vi "CRYPort Number Finder.vi"(9 "N interfs":i32=3, 10 "Interf settings":T1(array[cluster]), 11 "RS-232 type":enum16{"comm", "footswitch", "buzzer"}(ring)) -> (2 "Such a port exists":bool, 3 "Port (LV)":i32)   [LabVIEW 2013]
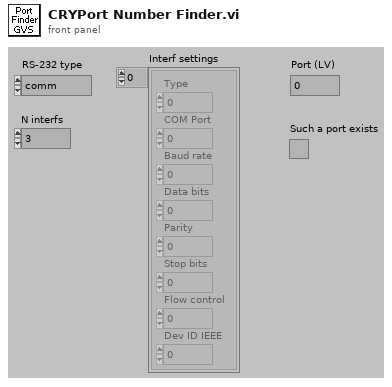
[diagram p1: front panel]
types:
  T1 = cluster{"Type":u16, "COM Port":u8, "Baud rate":u32, "Data bits":u32, "Parity":u16, "Stop bits":u16, "Flow control":u16, "Dev ID IEEE":u8}[]
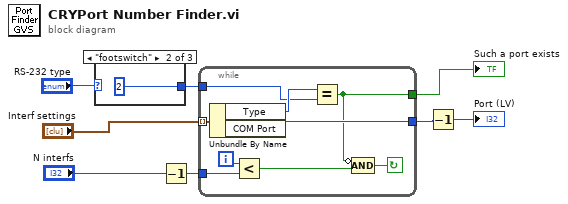
[diagram p0: block diagram]
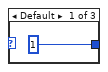
[diagram p2: hidden frame]
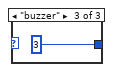
[diagram p3: hidden frame]
diagram:
  n1 = case shown="\"footswitch\"" "RS-232 type" {
    tunnel: [1 2 3] -> w6
    frame Default {
    }
    frame "footswitch" {
    }
    frame "buzzer" {
    }
  }
  n2 = Decrement(x="N interfs") -> (x-1=w8:i32)
  n3 = while {
    tunnel: w6 -> [w12]
    tunnel: [w13] -> w3
    tunnel: [w14] -> w2
    tunnel: w8 -> [w20]
    tunnel: "Interf settings" -> [w16] mode=indexing
    i -> [w19]
    stop <- w15 continue-if-true
    n4 = Unbundle By Name(w16) -> ("Type"=w17:u16, "COM Port"=w14:u8)
    n5 = Less?(x=w19, y=w20) -> (x < y?=w18:bool)
    n6 = Equal?(x=w17, y=w12) -> (x = y?=w13:bool)
    n7 = Compound Arithmetic op=AND(invert w13, w18) -> (w15:bool)
  }
  "Such a port exists" <- w3
  n8 = Decrement(x=w2) -> (x-1=→"Port (LV)":u8)
